vi "EnableDisable.vi"(7 "Command":T1(ring), 8 "error in":errorcluster, 11 "Array":refnum<vi>[](array[refnum])) -> (0 "error out":errorcluster)   [LabVIEW 2013]
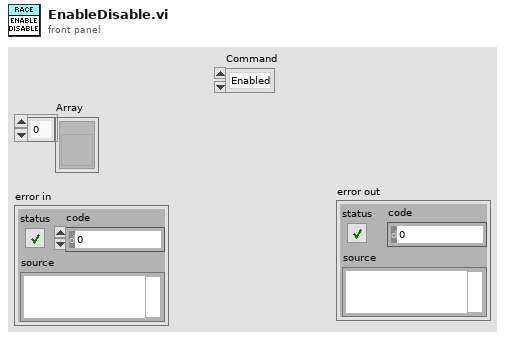
[diagram p1: front panel]
types:
  T1 = enum8{"Enabled", "Disabled", "Disabled and Grayed Out"}
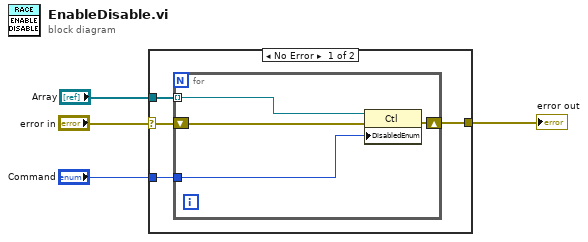
[diagram p0: block diagram]
diagram:
  n1 = case shown="No Error" "error in" {
    selector: "error in" -> [w5 w13]
    tunnel: [w8 w13] -> w4
    tunnel: "Command" -> [w7 _]
    tunnel: "Array" -> [w6 _]
    frame No Error {
      n2 = for {
        tunnel: w6 -> [w12] mode=indexing
        tunnel: w7 -> [w9]
        shift-right: [w10] -> w8
        shift-left: w5 -> [w11]
        n3 = property on="Property Node" class="Ctl"(reference=w12, error in=w11, "DisabledEnum"=w9) -> (error out=w10:errorcluster)  [unwired: 1 out]
      }
    }
    frame Error {
    }
  }
  "error out" <- w4
